vi "_PC_SaveFile updGraphProp.vi"(8 "error in (no error)":errorcluster, 11 "XY Graph in":refnum<vi>) -> (0 "error out":errorcluster, 3 "XY Graph out":refnum<vi>)   [LabVIEW 2018]
uses:
  <vilib>/Utility/miscctls.llb/LVMajorAndMinorColorsTypeDef.ctl
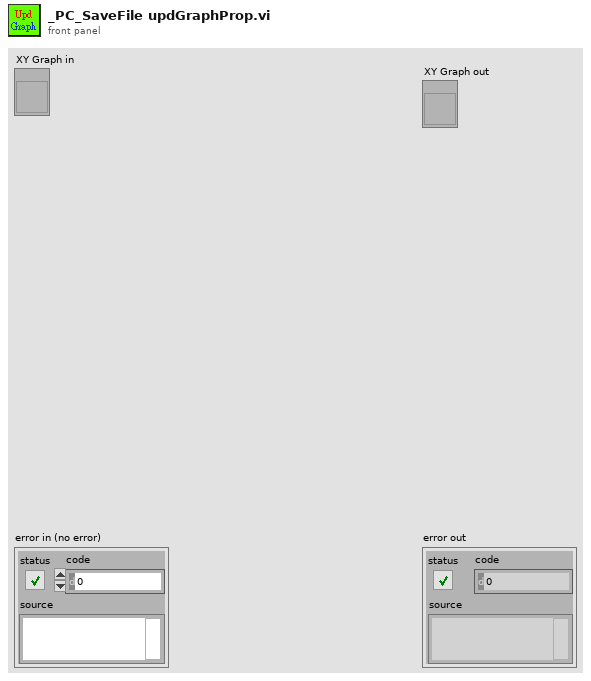
[diagram p1: front panel]
types:
  T1 = typedef "LVMajorAndMinorColorsTypeDef.ctl" = cluster{"Major Color":u32, "Minor Color":u32}
  T2 = cluster{"BGColor":u32, "GridX":bool, "GridY":bool, "LineColorArray":u32[], "LineWidthArray":u8[]}
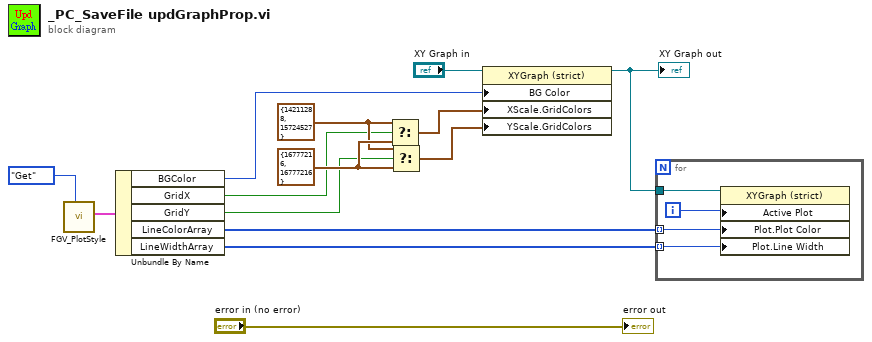
[diagram p0: block diagram]
diagram:
  w14 = T1 {"Major Color"=16777216, "Minor Color"=16777216} ("X Scale.Grid Colors")
  w13 = T1 {"Major Color"=14211288, "Minor Color"=15724527} ("X Scale.Grid Colors")
  n1 = call "FGV_PlotStyle.vi"("Function"=enum16{"Set", "Get"}."Get") -> ("Output Cluster"=w4:T2)  [unwired: 9 in, 1 out]
  n2 = Unbundle By Name(w4) -> ("BGColor"=w8:u32, "GridX"=w12:bool, "GridY"=w11:bool, "LineColorArray"=w6:u32[], "LineWidthArray"=w5:u8[])
  n3 = Select(t=w13, s=w12, f=w14) -> (s? t:f=w10:T1)
  n4 = Select(t=w13, s=w11, f=w14) -> (s? t:f=w9:T1)
  n5 = property class="XYGraph (strict)"(reference="XY Graph in", "BG Color"=w8, "XScale.GridColors"=w10, "YScale.GridColors"=w9) -> (reference out=w3:refnum<vi>)  [unwired: 1 in, 1 out]
  "XY Graph out" <- w3
  n6 = for {
    tunnel: w3 -> [w18]
    tunnel: w6 -> [w16] mode=indexing
    tunnel: w5 -> [w15] mode=indexing
    i -> [w17]
    n7 = property class="XYGraph (strict)"(reference=w18, "Active Plot"=w17, "Plot.Plot Color"=w16, "Plot.Line Width"=w15) -> ()  [unwired: 1 in, 2 out]
  }
  "error out" <- "error in (no error)"
